vi "FourBarDown.vi"(11 "Effort":dbl format="%#_13g") -> ()   [LabVIEW 2018]
uses:
  <vilib>/Rock Robotics/WPI/ThirdParty/Phoenix-LabVIEW/Motor Controller/Controls/CTRE_Phoenix_MotorControl_ControlMode.ctl
panel:
  in  "Min Joystick":dbl=0.3 format="%#_13g"
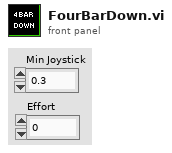
[diagram p1: front panel]
types:
  T1 = typedef "CTRE_Phoenix_MotorControl_ControlMode.ctl" = u16
  T2 = typedef "WPI_SwitchDevRef.ctl" = cluster{"DevStatus":errorcluster, "DIO Channel":T3, "CntIndex":T4, "Normally Closed":bool}
  T3 = typedef "FPGA_DIOChannel.ctl" = enum8{"DIO 0", "DIO 1", "DIO 2", "DIO 3", "DIO 4", "DIO 5", "DIO 6", "DIO 7", "DIO 8", "DIO 9", "DIO MXP 0", "DIO MXP 1", "DIO MXP 2", "DIO MXP 3", "DIO MXP 4", "DIO MXP 5", "DIO MXP 6", "DIO MXP 7", "DIO MXP 8", "DIO MXP 9", "DIO MXP 10", "DIO MXP 11", "DIO MXP 12", "DIO MXP 13", "DIO MXP 14", "DIO MXP 15", "SPI Port CS1", "SPI Port CS2", "SPI Port CS3", "SPI Port MISO", "SPI Port MOSI", "Invalid"}
  T4 = typedef "FPGA_CounterCtrSystemIndex.ctl" = enum8{"Ctr 0", "Ctr 1", "Ctr 2", "Ctr 3", "Ctr 4", "Ctr 5", "Ctr 6", "Ctr 7", "Invalid"}
  T5 = typedef "WPI_MotorControlDeviceRef.ctl" = cluster{"DeviceStatus":errorcluster, "Type":T6, "PWM":cluster{"PWM Channel":T7, "DeadBand":T8}, "CAN":cluster{"Device Number":u8, "SetOutput VI Ref":variant, "GetOutput VI Ref":variant, "Enable VI Ref":variant, "Disable VI Ref":variant, "Data":variant}, "Invert":bool, "DIO PWM":cluster{"PWM \"Enable\" Channel":T7, "DIOChannel":T3, "PWM Rate":dbl}}
  T6 = typedef "WPI_MotorControlType.ctl" = enum16{"PWM", "CAN", "DIO PWM"}
  T7 = typedef "FPGA_DIOPWMChannel.ctl" = enum8{"PWM 0", "PWM 1", "PWM 2", "PWM 3", "PWM 4", "PWM 5", "PWM 6", "PWM 7", "PWM 8", "PWM 9", "PWM MXP 0", "PWM MXP 1", "PWM MXP 2", "PWM MXP 3", "PWM MXP 4", "PWM MXP 5", "PWM MXP 6", "PWM MXP 7", "PWM MXP 8", "PWM MXP 9", "Invalid"}
  T8 = typedef "WPI_PWMDeadband.ctl" = cluster{"Name":string, "maxPositivePwm":i32, "minPositivePwm":i32, "centerPwm":i32, "maxNegativePwm":i32, "minNegativePwm":i32, "angularRange":u16}
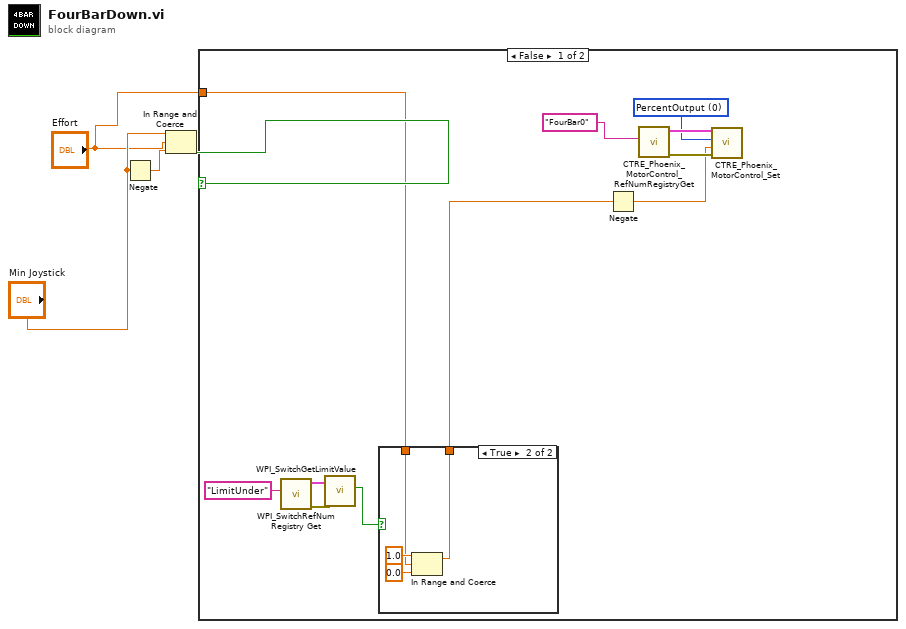
[diagram p0: block diagram]
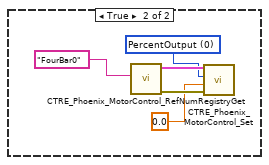
[diagram p3: hidden frame]
diagram:
  n1 = Negate(x="Min Joystick") -> (-x=w3:dbl)
  n2 = In Range and Coerce(upper limit="Min Joystick", x="Effort", lower limit=w3) -> (In Range?=w2:bool)  [unwired: 1 out]
  n3 = case shown="False" w2 {
    tunnel: "Effort" -> [w6 _]
    frame False {
      w13 = T1 0 items=["PercentOutput"=0, "Position"=1, "Velocity"=2, "Current"=3, "Follower"=5, "MotionProfile"=6, "MotionMagic"=7, "MotionMagicArc"=8, "MotionProfileArc"=10, "Disabled"=15] ("Control Mode")
      n4 = call <vilib>:"WPI_SwitchRefNum Registry Get.vi"("refnum name"="LimitUnder") -> ("error out"=w9:errorcluster, "SwitchDevRef"=w10:T2)  [unwired: 9 in]
      n5 = call <vilib>:"WPI_SwitchGetLimitValue.vi"("error in (no error)"=w9, "SwitchDevRef"=w10) -> ("Switch Pressed"=w7:bool)  [unwired: 7 in, 2 out]
      n6 = case shown="True" w7 {
        tunnel: [w16 w18] -> w5
        tunnel: w6 -> [w16 w17]
        frame False {
        }
        frame True {
          n7 = In Range and Coerce(upper limit=1.0, x=w17, lower limit=0.0) -> (coerced(x)=w18:dbl)  [unwired: 1 out]
        }
      }
      n8 = Negate(x=w5) -> (-x=w11:dbl)
      n9 = call <vilib>:"CTRE_Phoenix_MotorControl_RefNumRegistryGet.vi"("refnum name"="FourBar0") -> ("error out"=w14:errorcluster, "PhoenixMotorControlDevRef"=w15:T5)  [unwired: 9 in]
      n10 = call <vilib>:"CTRE_Phoenix_MotorControl_Set.vi"("error in (no error)"=w14, "Output"=w11, "Control Mode"=w13, "PhoenixMotorControlDevRef"=w15) -> ()  [unwired: 6 in, 2 out]
    }
    frame True {
      w22 = T1 0 items=["PercentOutput"=0, "Position"=1, "Velocity"=2, "Current"=3, "Follower"=5, "MotionProfile"=6, "MotionMagic"=7, "MotionMagicArc"=8, "MotionProfileArc"=10, "Disabled"=15] ("Control Mode")
      n11 = call <vilib>:"CTRE_Phoenix_MotorControl_RefNumRegistryGet.vi"("refnum name"="FourBar0") -> ("error out"=w25:errorcluster, "PhoenixMotorControlDevRef"=w24:T5)  [unwired: 9 in]
      n12 = call <vilib>:"CTRE_Phoenix_MotorControl_Set.vi"("error in (no error)"=w25, "Output"=0.0, "Control Mode"=w22, "PhoenixMotorControlDevRef"=w24) -> ()  [unwired: 6 in, 2 out]
    }
  }
